vi "Read TC.vi"(0 "read buffer":string, 11 "Error In":errorcluster) -> (4 "Temp (C)":dbl, 6 "On/Off Actual":bool, 8 "On/Off Set":bool, 10 "Temp Set Point (C)":i32, 15 "Error Out":errorcluster)   [LabVIEW 2015]
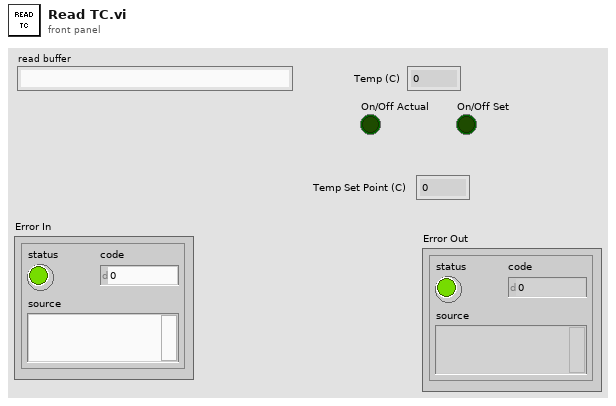
[diagram p1: front panel]
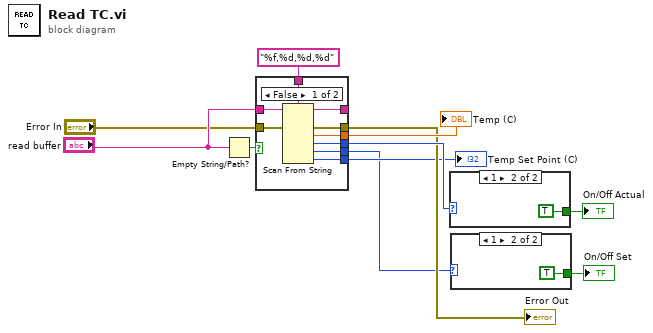
[diagram p0: block diagram]
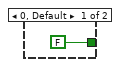
[diagram p2: hidden frame]
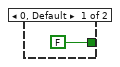
[diagram p3: hidden frame]
diagram:
  n1 = Empty String/Path?(string/path="read buffer") -> (empty?=w10:bool)
  n2 = case shown="False" w10 {
    tunnel: "read buffer" -> [w20 w22]
    tunnel: "%f,%d,%d,%d" ("format string") -> [w19 _]
    tunnel: [w18 w22] -> _
    tunnel: [w17 _] -> w8
    tunnel: [w16 _] -> w1
    tunnel: [w15 _] -> w7
    tunnel: [w14 w21] -> w5
    tunnel: "Error In" -> [w13 w21]
    tunnel: [w12 _] -> w2
    frame False {
      n3 = Scan From String(format string=w19, input string=w20, error in=w13) -> (remaining string=w18:string, error out=w14:errorcluster, output 1=w17:dbl, output 2=w15:i32, output 3=w16:i32, output 4=w12:i32)  [unwired: 5 in, 1 out]
    }
    frame True {
    }
  }
  "Temp (C)" <- w8
  "Temp Set Point (C)" <- w2
  "Error Out" <- w5
  n4 = case shown="1" w7 {
    tunnel: [FALSE TRUE] -> w6
    frame 0, Default {
    }
    frame 1 {
    }
  }
  "On/Off Actual" <- w6
  n5 = case shown="1" w1 {
    tunnel: [FALSE TRUE] -> w3
    frame 0, Default {
    }
    frame 1 {
    }
  }
  "On/Off Set" <- w3
